vi "Antonia_trend_max_min_najnowsze.vi"() -> ()   [LabVIEW 2025]
uses:
  <vilib>/Instr/_visa.llb/VISA Flush IO Buffer Mask.ctl
  <vilib>/Analysis/baseanly.llb/Mean (DBL).vi
  <vilib>/Utility/error.llb/Trim Whitespace One-Sided.vi
  <vilib>/Instr/_visa.llb/VISA Configure Serial Port (Instr).vi
  <vilib>/Analysis/NI_AALBase.lvlib
panel:
  in  "Tab Control":T1(tab)
  in  "Próg trendu - temp":dbl
  out "Temperatura średnia 5 próbek [C]":dbl
  out "Thermometer":dbl(slide) scale=0.0..100.0
  out "Temperatura wykres":dbl(graph)
  out "Temperatura liczba":dbl
  out "Temperatura max [C]":dbl
  out "Temperatura min[C]":dbl
  out "Temperatura średnia[C]":dbl
  out "TREND - TEMP":enum16{"STABILNY", "WZROST", "SPADEK"}(ring)
  in  "Próg trendu":dbl
  out "Wilgotność średnia 5 próbek [%]":dbl
  out "Wilgotność wykres":dbl(graph)
  out "Tank":dbl(slide) scale=0.0..100.0
  out "wilgotność liczba":dbl
  out "Wilgotnosc max [%]":dbl
  out "Wilogtność min [%]":dbl
  out "Wilgotność średnia[%]":dbl
  out "Trend":enum16{"STABILNY", "WZROST", "SPADEK"}(ring)
  out "Bardzo Suche":bool
  out "Punkt Rosy":dbl format="%#_4g"
  out "Indeks ciepła":dbl format="%#_4g"
  out "Suche":bool
  out "Komfort":bool
  out "Wilgotno":bool
  out "Bardzo Wilgotno":bool
  out "Komfort":bool
  out "Uwaga":bool
  out "Duża Ostrożność":bool
  out "Niebezpieczne":bool
  out "Ekstremalnie niebezpieczne":bool
  out "max Punkt Rosy":dbl
  out "min Punkt Rosy":dbl
  out "max Indeks ciepła":dbl
  out "min Indeks ciepła":dbl
  out "wyświetlanie danych":string
  out "Czy dziła whlie":i32
  out "numeric - start/stop":dbl
  in  "START/STOP":bool
  out "wyświetlanie danych 2":string
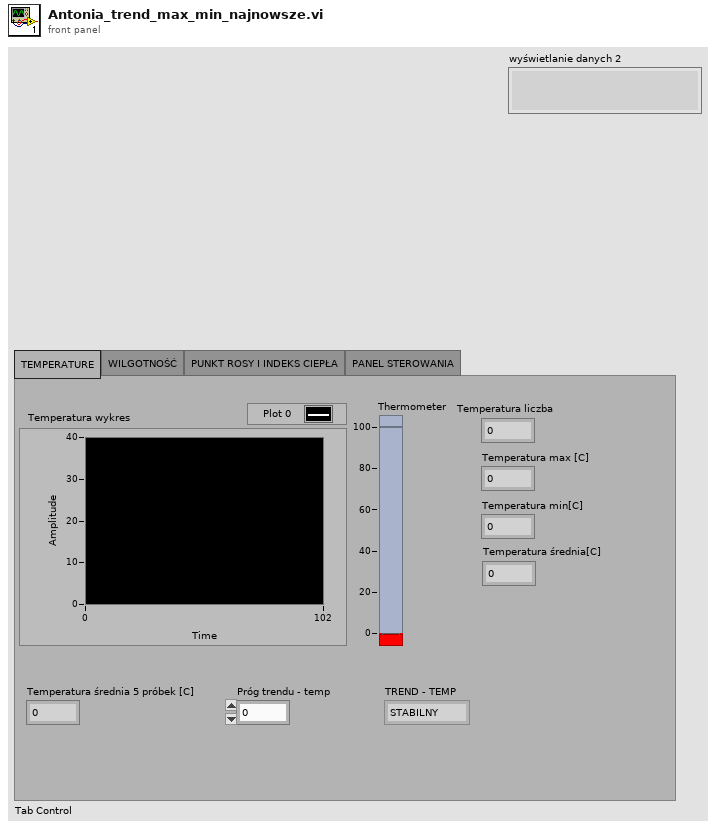
[diagram p1: front panel]
types:
  T1 = enum32{"TEMPERATURE", "WILGOTNOŚĆ", "PUNKT ROSY I INDEKS CIEPŁA", "PANEL STEROWANIA"}
  T2 = typedef "VISA Flush IO Buffer Mask.ctl" = u16
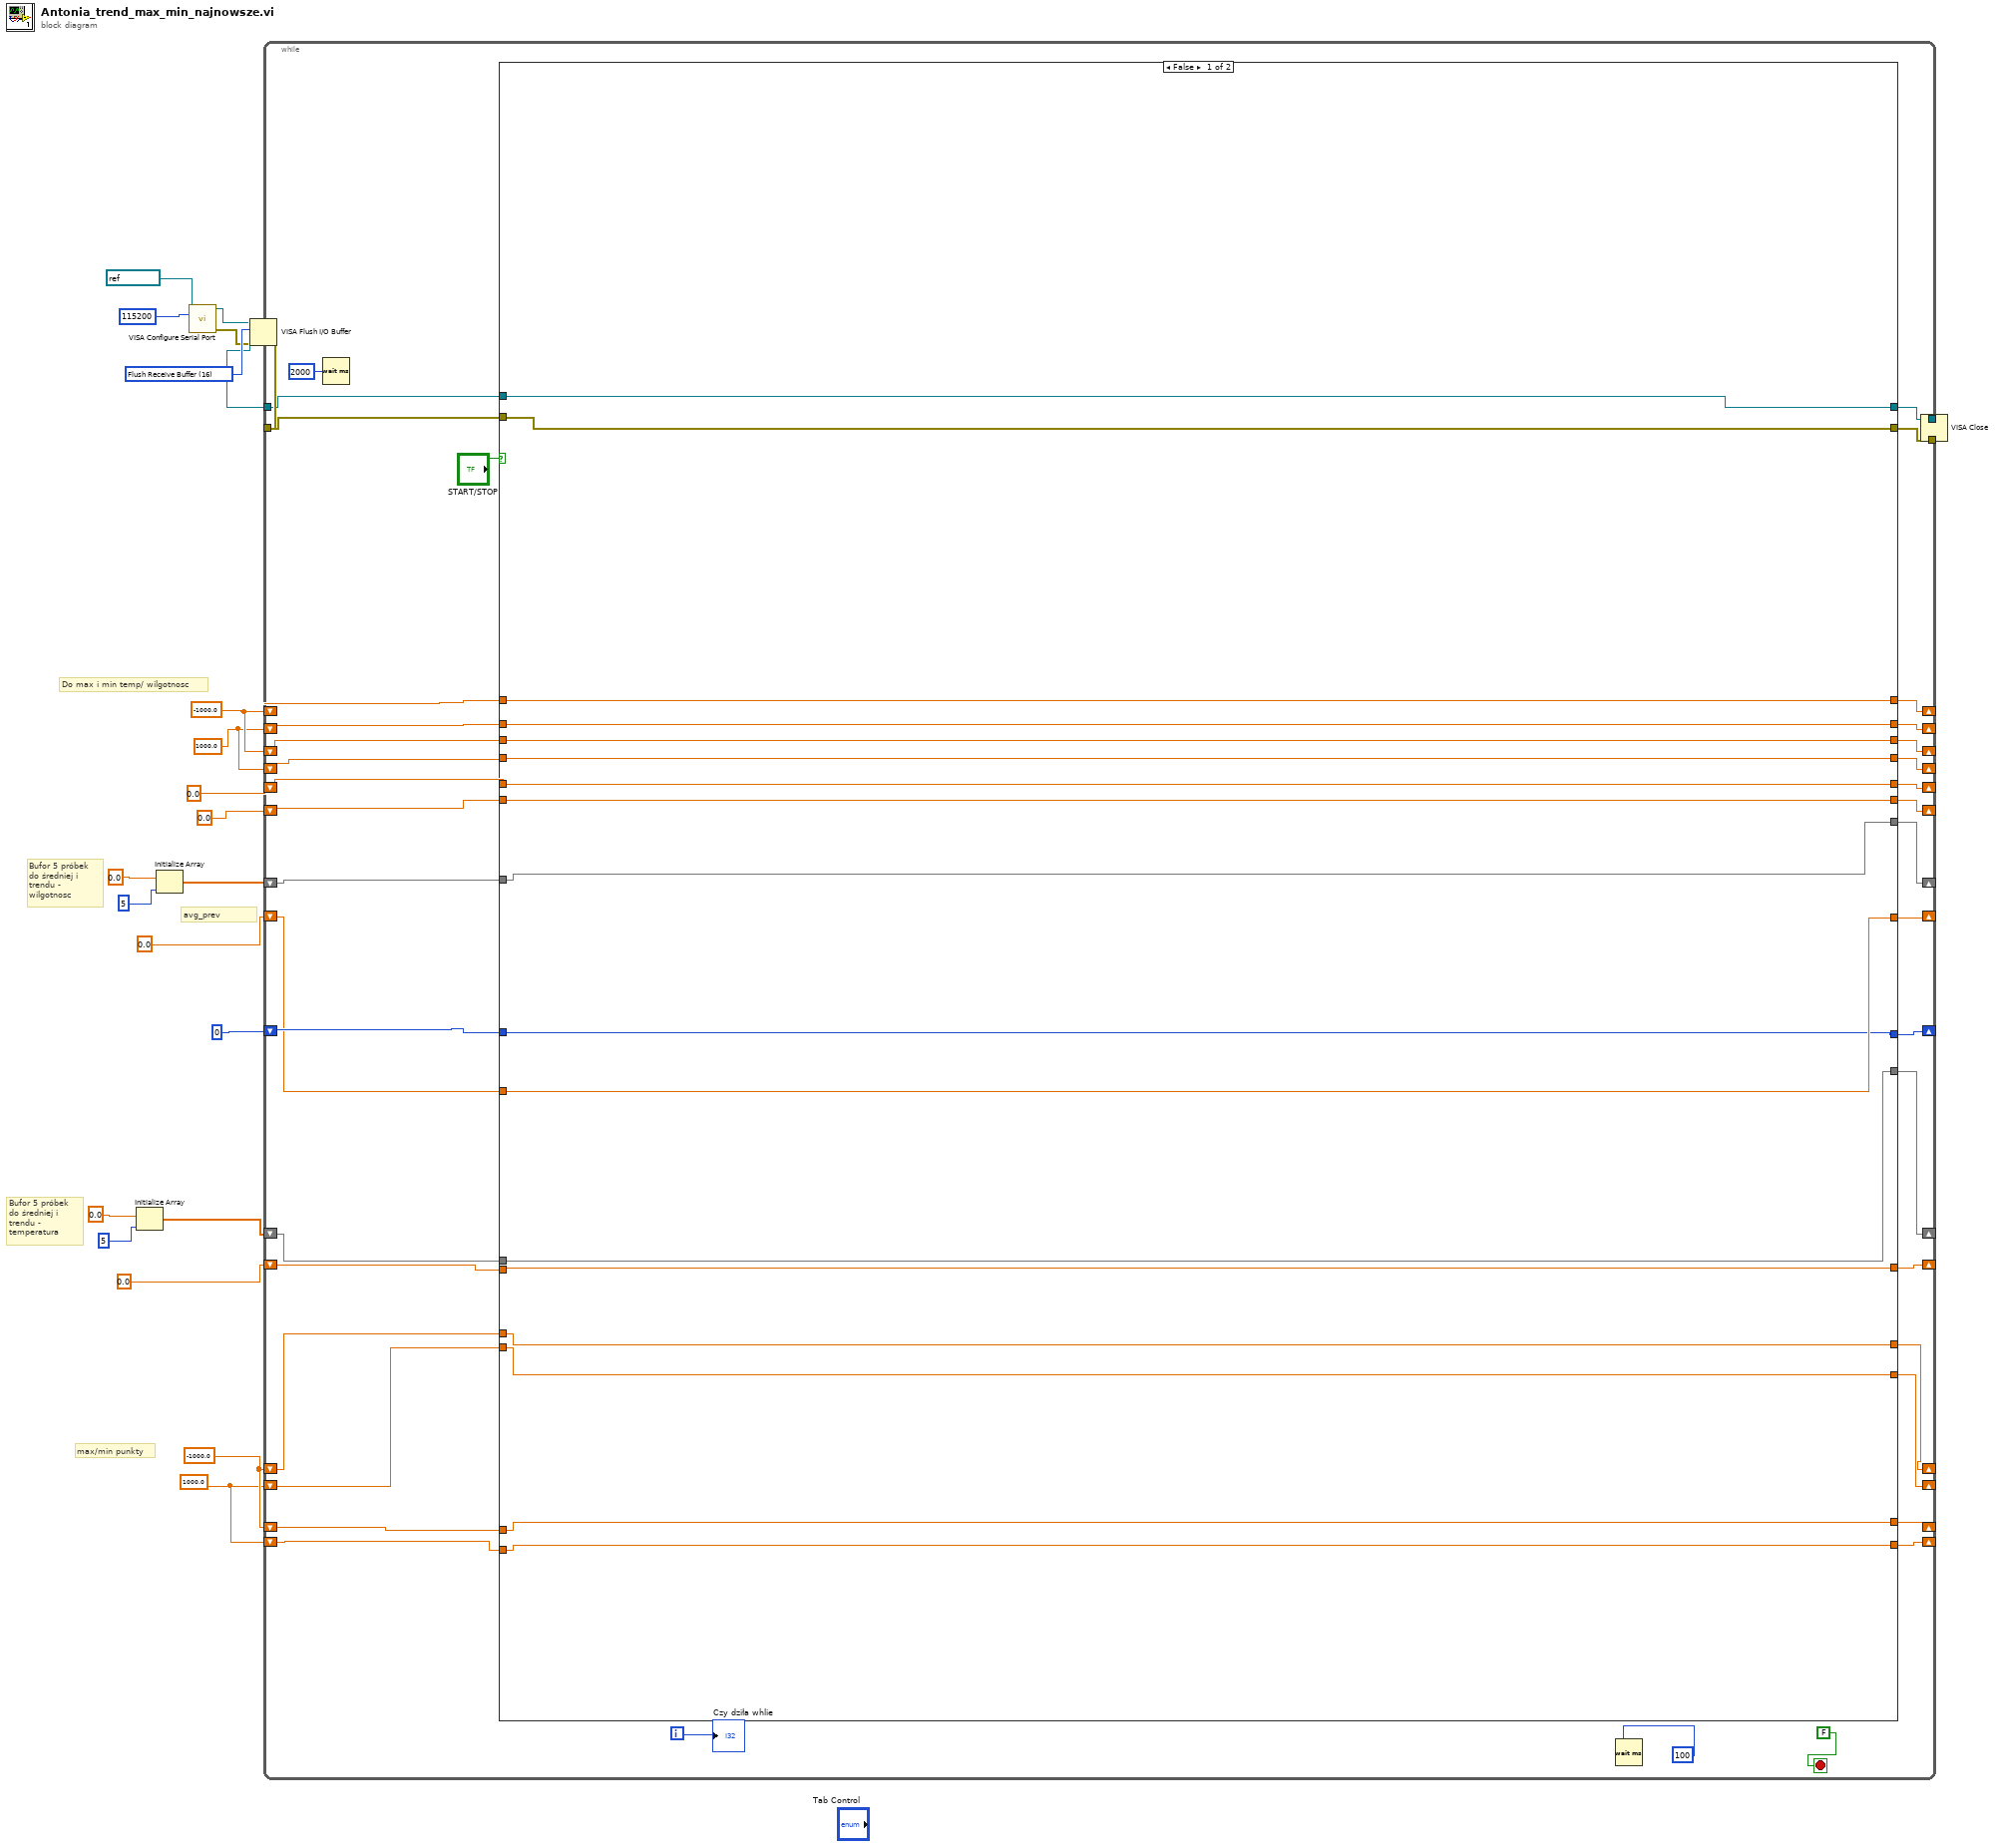
[diagram p0: block diagram]
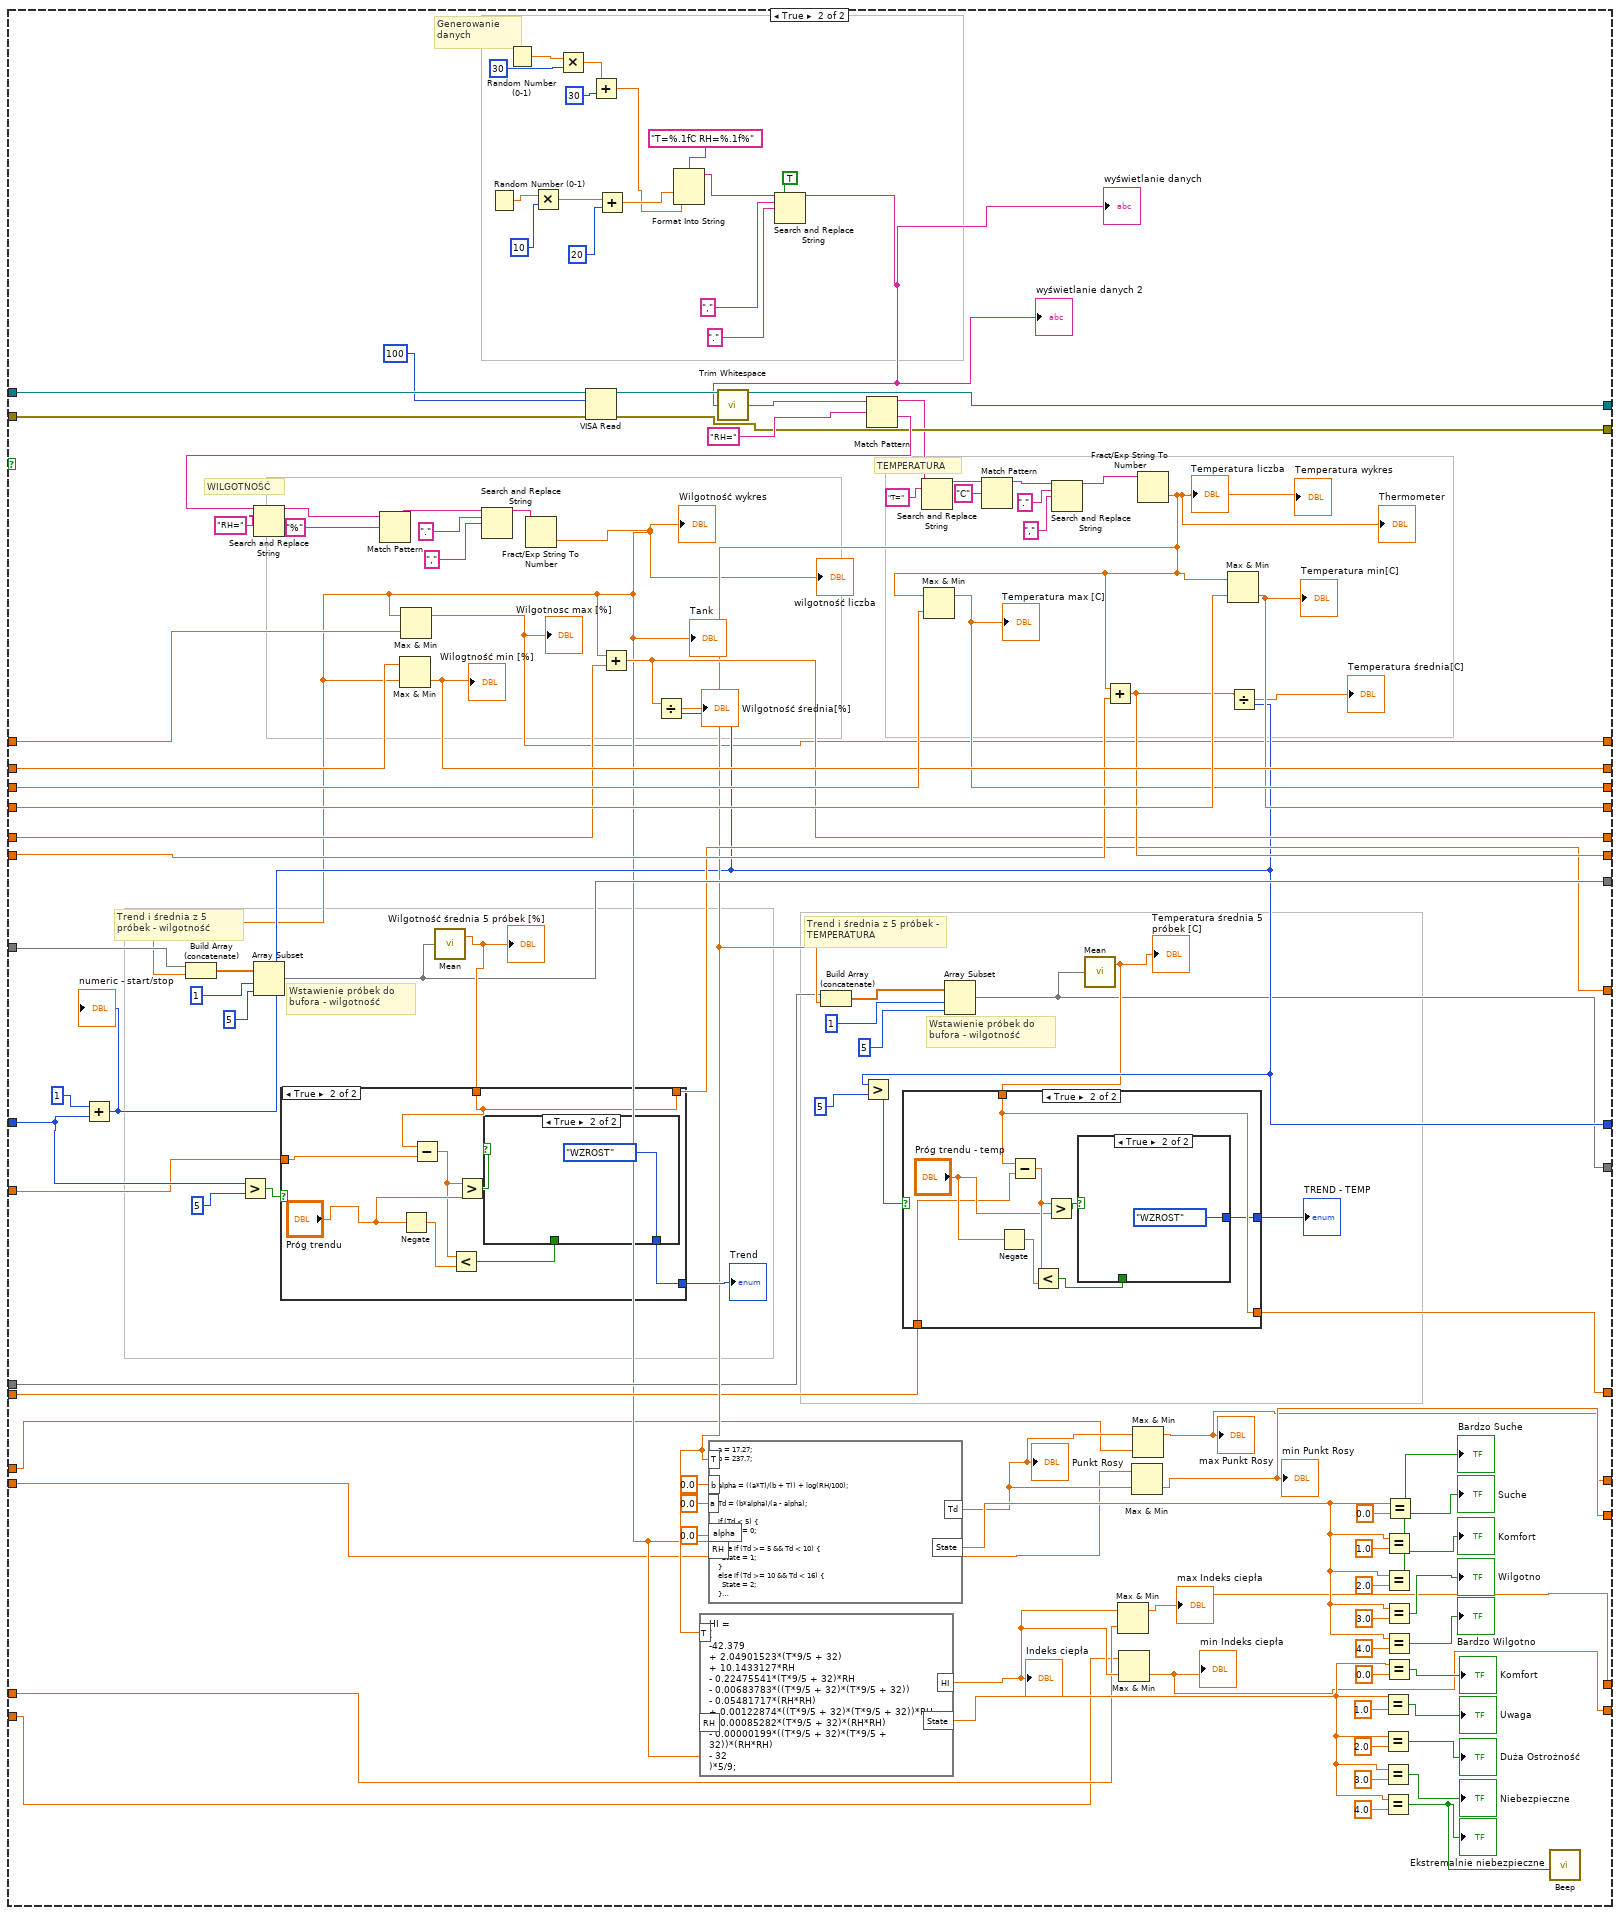
[diagram p2: hidden frame]
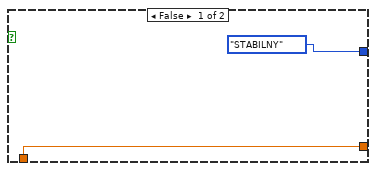
[diagram p3: hidden frame]
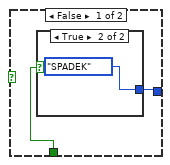
[diagram p4: hidden frame]
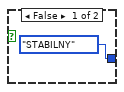
[diagram p5: hidden frame]
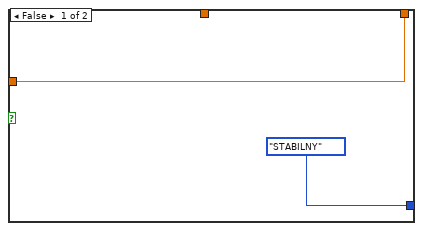
[diagram p6: hidden frame]
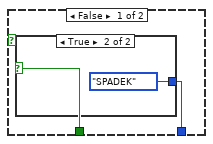
[diagram p7: hidden frame]
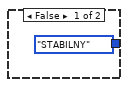
[diagram p8: hidden frame]
diagram:
  w1 = 1000.0
  w2 = -1000.0
  w3 = 1000.0
  w4 = -1000.0
  w25 = T2 16 items=["Flush Receive Buffer"=16, "Write Transmit Buffer to Device"=32, "Flush Receive Buffer (No I/O)"=64, "Flush Transmit Buffer"=128] ("Mask")
  # "max/min punkty"
  # "Do max i min temp/ wilgotnosc"
  # "Bufor 5 próbek do średniej i trendu - temperatura"
  # "avg_prev"
  # "Bufor 5 próbek do średniej i trendu - wilgotnosc"
  n1 = Initialize Array(0.0, 5) -> (w6:dbl[])
  n2 = Initialize Array(0.0, 5) -> (w13:dbl[])
  n3 = call-poly "VISA Configure Serial Port"("VISA resource name"=refnum<visa-resource-name> "COM7", "baud rate (9600)"=u32 115200) -> ("VISA resource name out"=w20:refnum<visa-resource-name>, "error out"=w19:errorcluster)  [unwired: 12 in]
  n4 = VISA Flush I/O Buffer(VISA resource name=w20, mask (16)=w25, error in (no error)=w19) -> (VISA resource name out=w23:refnum<visa-resource-name>, error out=w22:errorcluster)
  n5 = while {
    shift-right: [w59] -> _
    shift-left: w4 -> [w43]
    shift-right: [w58] -> _
    shift-left: w3 -> [w62]
    shift-right: [w57] -> _
    shift-left: w4 -> [w61]
    shift-right: [w56] -> _
    shift-left: w3 -> [w60]
    shift-right: [w52] -> _
    shift-left: 0.0 -> [w55]
    shift-right: [w53] -> _
    shift-left: 0.0 -> [w54]
    shift-right: [w38] -> _
    shift-left: 0 -> [w49]
    tunnel: [w47] -> w24
    tunnel: w23 -> [w46]
    tunnel: w22 -> [w45]
    tunnel: [w44] -> w21
    shift-right: [w42] -> _
    shift-left: w13 -> [w41]
    shift-right: [w40] -> _
    shift-left: 0.0 -> [w39]
    shift-right: [w34] -> _
    shift-left: w6 -> [w37]
    shift-right: [w35] -> _
    shift-left: 0.0 -> [w36]
    shift-right: [w30] -> _
    shift-left: w2 -> [w33]
    shift-right: [w31] -> _
    shift-left: w1 -> [w32]
    shift-right: [w26] -> _
    shift-left: w2 -> [w29]
    shift-right: [w27] -> _
    shift-left: w1 -> [w28]
    i -> [w51]
    stop <- FALSE stop-if-true
    n6 = case shown="False" "START/STOP" {
      tunnel: w43 -> [w80 w163]
      tunnel: w62 -> [w79 w162]
      tunnel: w61 -> [w78 w161]
      tunnel: w60 -> [w77 w160]
      tunnel: [w80 w91] -> w59
      tunnel: [w79 w159] -> w58
      tunnel: [w78 w158] -> w57
      tunnel: [w77 w157] -> w56
      tunnel: w55 -> [w76 w156]
      tunnel: w54 -> [w75 w155]
      tunnel: [w75 w154] -> w53
      tunnel: [w76 w145] -> w52
      tunnel: w49 -> [w70 w112]
      tunnel: [w73 w151] -> w47
      tunnel: w46 -> [w73 w148]
      tunnel: w45 -> [w74 w150]
      tunnel: [w74 w149] -> w44
      tunnel: w41 -> [w71 w117]
      tunnel: [w71 w107] -> w42
      tunnel: [w72 w106] -> w40
      tunnel: w39 -> [w72 w110]
      tunnel: [w70 w99] -> w38
      tunnel: w37 -> [w69 w101]
      tunnel: w36 -> [w68 w97]
      tunnel: [w68 w95] -> w35
      tunnel: [w69 w94] -> w34
      tunnel: w33 -> [w65 w89]
      tunnel: w32 -> [w64 w88]
      tunnel: [w64 w87] -> w31
      tunnel: [w65 w86] -> w30
      tunnel: w29 -> [w67 w84]
      tunnel: w28 -> [w66 w83]
      tunnel: [w66 w82] -> w27
      tunnel: [w67 w81] -> w26
      frame False {
      }
      frame True {
        # "Trend i średnia z 5 próbek - TEMPERATURA"
        # "Wstawienie próbek do bufora - wilgotność"
        # "Trend i średnia z 5 próbek - wilgotność"
        # "Wstawienie próbek do bufora - wilgotność"
        # "Generowanie danych"
        # "WILGOTNOŚĆ"
        # "TEMPERATURA"
        n7 = Add(x=1, y=w112) -> (x+y=w99:i32)
        "numeric - start/stop" <- w99
        n8 = Greater?(x=w112, y=5) -> (0:w111:bool)
        n9 = Random Number (0-1)() -> (number: 0 to 1=w175:dbl)
        n10 = Random Number (0-1)() -> (number: 0 to 1=w177:dbl)
        n11 = Multiply(x=w175, y=10) -> (x*y=w176:dbl)
        n12 = Multiply(x=w177, y=30) -> (x*y=w178:dbl)
        n13 = VISA Read(VISA resource name=w148, byte count=u32 100, error in (no error)=w150) -> (VISA resource name out=w151:refnum<visa-resource-name>, error out=w149:errorcluster)  [unwired: 2 out]
        n14 = Add(x=w178, y=30) -> (x+y=w164:dbl)
        n15 = Add(x=w176, y=20) -> (x+y=w165:dbl)
        n16 = Format Into String(format string="T=%.1fC RH=%.1f%", w165, w164) -> (resulting string=w166:string)  [unwired: 2 in, 1 out]
        n17 = Search and Replace String(replace all?=TRUE, input string=w166, search string=",", replace string=".") -> (result string=w118:string)  [unwired: 4 in, 3 out]
        "wyświetlanie danych" <- w118
        "wyświetlanie danych 2" <- w118
        n18 = call <vilib>:"Trim Whitespace.vi"("string"=w118) -> ("trimmed string"=w188:string)  [unwired: 1 in]
        n19 = Greater?(x=w99, y=5) -> (0:w98:bool)
        n20 = Match Pattern(string=w188, regular expression="RH=") -> (before substring=w146:string, after substring=w192:string)  [unwired: 1 in, 2 out]
        n21 = Search and Replace String(input string=w192, search string="RH=") -> (result string=w193:string)  [unwired: 6 in, 3 out]
        n22 = Match Pattern(string=w193, regular expression="%") -> (before substring=w194:string)  [unwired: 1 in, 3 out]
        n23 = Search and Replace String(input string=w194, search string=".", replace string="," ("replace string (\"\")")) -> (result string=w195:string)  [unwired: 5 in, 3 out]
        n24 = Fract/Exp String To Number(string=w195) -> (number=w92:dbl)  [unwired: 3 in, 1 out]
        "Wilgotność wykres" <- w92
        "wilgotność liczba" <- w92
        "Tank" <- w92
        n25 = Build Array (concatenate)(w117, w92) -> (w116:dbl[])
        n26 = Array Subset(array=w116, index=1, length=5) -> (w107:dbl[])
        n27 = Max & Min(x=w162, y=w92) -> (min(x,y)=w159:dbl)  [unwired: 1 out]
        "Wilogtność min [%]" <- w159
        n28 = Max & Min(x=w92, y=w163) -> (max(x,y)=w91:dbl)  [unwired: 1 out]
        "Wilgotnosc max [%]" <- w91
        n29 = call-poly <vilib>:"Mean.vi"("X"=w107) -> ("mean"=w109:dbl)  [unwired: 1 out]
        "Wilgotność średnia 5 próbek [%]" <- w109
        n30 = case shown="True" w111 {
          tunnel: w110 -> [w212 w220]
          tunnel: w109 -> [_ w213]
          tunnel: [enum16{"STABILNY", "WZROST", "SPADEK"}."STABILNY" ("Trend") w214] -> w108
          tunnel: [w212 w213] -> w106
          frame False {
          }
          frame True {
            n31 = Negate(x="Próg trendu") -> (-x=w218:dbl)
            n32 = Subtract(x=w213, y=w220) -> (x-y=w217:dbl)
            n33 = Less?(x=w217, y=w218) -> (x < y?=w215:bool)
            n34 = Greater?(x=w217, y="Próg trendu") -> (0:w216:bool)
            n35 = case shown="True" w216 {
              tunnel: w215 -> [w222 _]
              tunnel: [w221 enum16{"STABILNY", "WZROST", "SPADEK"}."WZROST" ("Trend")] -> w214
              frame False {
                n36 = case shown="True" w222 {
                  tunnel: [enum16{"STABILNY", "WZROST", "SPADEK"}."STABILNY" ("Trend") enum16{"STABILNY", "WZROST", "SPADEK"}."SPADEK" ("Trend")] -> w221
                  frame False {
                  }
                  frame True {
                  }
                }
              }
              frame True {
              }
            }
          }
        }
        "Trend" <- w108
        n37 = Add(x=w92, y=w156) -> (x+y=w145:dbl)
        n38 = Divide(x=w145, y=w99) -> (x/y=→"Wilgotność średnia[%]":dbl)
        n39 = Search and Replace String(input string=w146, search string="T=" ("replace string (\"\")")) -> (result string=w189:string)  [unwired: 6 in, 3 out]
        n40 = Match Pattern(string=w189, regular expression="C") -> (before substring=w190:string)  [unwired: 1 in, 3 out]
        n41 = Search and Replace String(input string=w190, search string=".", replace string="," ("replace string (\"\")")) -> (result string=w191:string)  [unwired: 5 in, 3 out]
        n42 = Fract/Exp String To Number(string=w191) -> (number=w102:dbl)  [unwired: 3 in, 1 out]
        "Temperatura wykres" <- w102
        "Temperatura liczba" <- w102
        "Thermometer" <- w102
        n43 = formula code="HI =\n(\n-42.379\n+ 2.04901523*(T*9/5 + 32)\n+ 10.1433127*RH\n- 0.22475541*(T*9/5 + 32)*RH\n- 0.00683783*((T*9/5 + 32)*(T*9/5 + 32))\n- 0.05481717*(RH*RH)\n+ 0.00122874*((T*9/5 + 32)*(T*9/5 + 32))*RH\n+ 0.00085282*(T*9/5 + 32)*(RH*RH)\n- 0.00000199*((T*9/5 + 32)*(T*9/5 + 32))*(RH*RH)\n- 32\n)*5/9;\n\n\nif (HI < 27) {\n  State = 0;\n}\nelse if (HI >= 27 && HI < 32) {\n  State = 1;\n}\nelse if (HI >= 32 && HI < 41) {\n  State = 2;\n}\nelse if (HI >= 41 && HI < 54) {\n  State = 3;\n}\nelse {\n  State = 4;\n}"("T"=w102, "RH"=w92) -> ("HI"=w85:dbl, "State"=w130:dbl)
        "Indeks ciepła" <- w85
        n44 = formula code="a = 17.27;\nb = 237.7;\n\n\nalpha = ((a*T)/(b + T)) + log(RH/100);\n\nTd = (b*alpha)/(a - alpha);\n\nif (Td < 5) {\n  State = 0;\n}\nelse if (Td >= 5 && Td < 10) {\n  State = 1;\n}\nelse if (Td >= 10 && Td < 16) {\n  State = 2;\n}\nelse if (Td >= 16 && Td < 20) {\n  State = 3;\n}\nelse {\n  State = 4;\n}"("T"=w102, "RH"=w92, "a"=0.0 ("input variable"), "b"=0.0 ("input variable"), "alpha"=0.0 ("input variable")) -> ("Td"=w90:dbl, "State"=w129:dbl)
        "Punkt Rosy" <- w90
        n45 = Build Array (concatenate)(w101, w102) -> (w105:dbl[])
        n46 = Max & Min(x=w102, y=w161) -> (max(x,y)=w158:dbl)  [unwired: 1 out]
        "Temperatura max [C]" <- w158
        n47 = Array Subset(array=w105, index=1, length=5) -> (w94:dbl[])
        n48 = call-poly <vilib>:"Mean.vi"("X"=w94) -> ("mean"=w96:dbl)  [unwired: 1 out]
        "Temperatura średnia 5 próbek [C]" <- w96
        n49 = case shown="True" w98 {
          tunnel: w97 -> [w197 w202]
          tunnel: w96 -> [_ w201]
          tunnel: [w197 w201] -> w95
          tunnel: [enum16{"STABILNY", "WZROST", "SPADEK"}."STABILNY" w198] -> w93
          frame False {
          }
          frame True {
            n50 = Negate(x="Próg trendu - temp") -> (-x=w205:dbl)
            n51 = Subtract(x=w201, y=w202) -> (x-y=w204:dbl)
            n52 = Less?(x=w204, y=w205) -> (x < y?=w199:bool)
            n53 = Greater?(x=w204, y="Próg trendu - temp") -> (0:w200:bool)
            n54 = case shown="True" w200 {
              tunnel: w199 -> [w207 _]
              tunnel: [w206 enum16{"STABILNY", "WZROST", "SPADEK"}."WZROST"] -> w198
              frame False {
                n55 = case shown="True" w207 {
                  tunnel: [enum16{"STABILNY", "WZROST", "SPADEK"}."STABILNY" enum16{"STABILNY", "WZROST", "SPADEK"}."SPADEK"] -> w206
                  frame False {
                  }
                  frame True {
                  }
                }
              }
              frame True {
              }
            }
          }
        }
        "TREND - TEMP" <- w93
        n56 = Add(x=w102, y=w155) -> (x+y=w154:dbl)
        n57 = Max & Min(x=w85, y=w84) -> (max(x,y)=w81:dbl)  [unwired: 1 out]
        "max Indeks ciepła" <- w81
        n58 = Max & Min(x=w83, y=w85) -> (min(x,y)=w82:dbl)  [unwired: 1 out]
        "min Indeks ciepła" <- w82
        n59 = Max & Min(x=w88, y=w90) -> (min(x,y)=w87:dbl)  [unwired: 1 out]
        "min Punkt Rosy" <- w87
        n60 = Max & Min(x=w90, y=w89) -> (max(x,y)=w86:dbl)  [unwired: 1 out]
        "max Punkt Rosy" <- w86
        n61 = Max & Min(x=w102, y=w160) -> (min(x,y)=w157:dbl)  [unwired: 1 out]
        "Temperatura min[C]" <- w157
        n62 = Divide(x=w154, y=w99) -> (x/y=→"Temperatura średnia[C]":dbl)
        n63 = Equal?(x=w130, y=1.0) -> (x = y?=→"Uwaga":bool)
        n64 = Equal?(x=w130, y=2.0) -> (x = y?=→"Duża Ostrożność":bool)
        n65 = Equal?(x=w130, y=3.0) -> (x = y?=→"Niebezpieczne":bool)
        n66 = Equal?(x=w130, y=4.0) -> (x = y?=w119:bool)
        "Ekstremalnie niebezpieczne" <- w119
        n67 = Equal?(x=w129, y=1.0) -> (x = y?=→"Suche":bool)
        n68 = Equal?(x=w129, y=2.0) -> (x = y?=→"Komfort":bool)
        n69 = Equal?(x=w129, y=3.0) -> (x = y?=→"Wilgotno":bool)
        n70 = Equal?(x=w129, y=4.0) -> (x = y?=→"Bardzo Wilgotno":bool)
        n71 = Equal?(x=w130, y=0.0) -> (x = y?=→"Komfort":bool)
        n72 = Equal?(x=w129, y=0.0) -> (x = y?=→"Bardzo Suche":bool)
        n73 = call <vilib>:"Beep.vi"("use system alert? (T)"=w119) -> ()  [unwired: 11 in]
      }
    }
    n74 = Wait (ms)(milliseconds to wait=u32 100) -> ()  [unwired: 1 out]
    "Czy dziła whlie" <- w51
  }
  n75 = Wait (ms)(milliseconds to wait=u32 2000) -> ()  [unwired: 1 out]
  n76 = VISA Close(VISA resource name=w24, error in (no error)=w21) -> ()  [unwired: 1 out]
